vi "Configure Math Expression (Binary Operation).vi"(7 "Operator (0: Add)":u16(ring) items=["Add", "Subtract", "Multiply", "Divide"], 8 "error in (no error)":errorcluster, 9 "Expression Input 2":string(combo), 10 "Expression Input 1":string(combo), 11 "VISA resource name":refnum<visa-resource-name>) -> (0 "error out":errorcluster, 2 "Expression Output":string, 3 "VISA resource name out":refnum<visa-resource-name>)   [LabVIEW 2015, in "Tektronix 7000 Series.lvlib"]
doc: "Creates a mathematical expression with two operands.\n\n<B>Note:</B> The TDS 5000 series will not support most unary functions or support nested functions without the math option installed."
uses:
  <instrlib>/Tektronix 7000 Series/Tektronix 7000 Series.lvlib
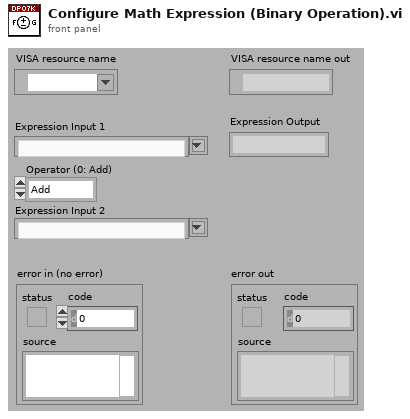
[diagram p1: front panel]
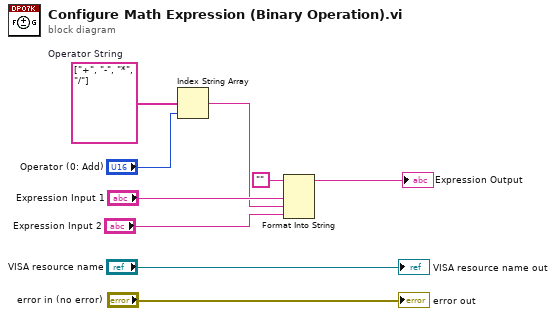
[diagram p0: block diagram]
diagram:
  w9 = string[] ["+", "-", "*", "/"]  # Operator String
  n1 = Index String Array(1:"Operator (0: Add)", 2:w9) -> (0:w5:string)  [unwired: 1 in]
  n2 = Format Into String(initial string="" ("Empty String Constant"), "Expression Input 1", w5, "Expression Input 2") -> (resulting string=→"Expression Output":string)  [unwired: 2 in, 1 out]
  "VISA resource name out" <- "VISA resource name"
  "error out" <- "error in (no error)"
